vi "OneBallAuton.vi"   [LabVIEW 2013]
uses:
  <vilib>/Rock Robotics/WPI/SafetyOutput/WPI_SafetyOutputConfigMenu.ctl
  <vilib>/Rock Robotics/WPI/Solenoid/WPI_SolenoidValue.ctl
  <vilib>/Rock Robotics/WPI/RobotDrive/WPI_RobotDriveGetSetRefNum.vi
  <vilib>/Rock Robotics/WPI/Solenoid/WPI_SolenoidSetEnum.vi
types:
  T1 = typedef "WPI_SafetyOutputConfigMenu.ctl" = enum16{"Enable", "Disable"}
  T2 = typedef "WPI_RobotDriveDevRef.ctl" = cluster{"DevStatus":errorcluster, "Motors[]":T3[], "Square Inputs":bool, "Max Output":dbl, "Isochronous":bool}
  T3 = typedef "WPI_MotorControlDeviceRef.ctl" = cluster{"DeviceStatus":errorcluster, "Type":enum16{"PWM", "CAN"}, "PWM":cluster{"Digital Module":T4, "PWM Channel":T5, "DeadBand":T6}, "CAN":cluster{"Device Number":u8, "Control Mode":T7, "Semaphore":T8, "Max Vout":dbl}, "Invert":bool, "TransformRef":T9, "InvTransformRef":T9}
  T4 = typedef "FPGA_TypedefDigitalModule.ctl" = enum16{"Digital Module 1", "Digital Module 2"}
  T5 = typedef "FPGA_DIOPWMChannel.ctl" = enum8{"PWM 1", "PWM 2", "PWM 3", "PWM 4", "PWM 5", "PWM 6", "PWM 7", "PWM 8", "PWM 9", "PWM 10", "Invalid"}
  T6 = typedef "WPI_PWMDeadband.ctl" = cluster{"Name":string, "maxPositivePwm":i32, "minPositivePwm":i32, "centerPwm":i32, "maxNegativePwm":i32, "minNegativePwm":i32, "angularRange":u16}
  T7 = typedef "WPI_CANJaguar_ControlMode.ctl" = enum8{"Percent VBus", "Current", "Speed", "Position", "Voltage"}
  T8 = typedef "Semaphore RefNum" = refnum<k1>
  T9 = typedef "WPI_PWMTransform_ConPane.ctl" = refnum<vi>
  T10 = typedef "WPI_SolenoidDevRef.ctl" = cluster{"DevStatus":errorcluster, "Solenoid Module":T11, "Forward Solenoid Channel":T12, "Reverse Solenoid Channel":T12}
  T11 = typedef "FPGA_TypedefSolenoidModule.ctl" = enum16{"Solenoid Module 1", "Solenoid Module 2"}
  T12 = typedef "WPI_SolenoidChannel.ctl" = enum8{"Solenoid 1", "Solenoid 2", "Solenoid 3", "Solenoid 4", "Solenoid 5", "Solenoid 6", "Solenoid 7", "Solenoid 8", "Invalid"}
  T13 = typedef "WPI_DigitalInputDevRef.ctl" = cluster{"DevStatus":errorcluster, "DIO Channel":T14, "Digital Module":T4}
  T14 = typedef "FPGA_DIOChannel.ctl" = enum8{"DIO 1", "DIO 2", "DIO 3", "DIO 4", "DIO 5", "DIO 6", "DIO 7", "DIO 8", "DIO 9", "DIO 10", "DIO 11", "DIO 12", "DIO 13", "DIO 14", "Invalid"}
  T15 = typedef "WPI_EncoderDevRef.ctl" = cluster{"DevStatus":errorcluster, "EncoderIndex":T16, "CounterIndex":T17, "DistancePerCount":dbl, "Decoding Type":T18}
  T16 = typedef "FPGA_EncoderIdx.ctl" = enum8{"Enc 0", "Enc 1", "Enc 2", "Enc 3", "Invalid"}
  T17 = typedef "FPGA_CounterCtrSystemIndex.ctl" = enum8{"Ctr 0", "Ctr 1", "Ctr 2", "Ctr 3", "Ctr 4", "Ctr 5", "Ctr 6", "Ctr 7", "Invalid"}
  T18 = typedef "WPI_EncoderType.ctl" = enum16{"1x", "2x", "4x"}
  T19 = typedef "WPI_SolenoidValue.ctl" = enum16{"Off", "On", "Forward", "Reverse"}
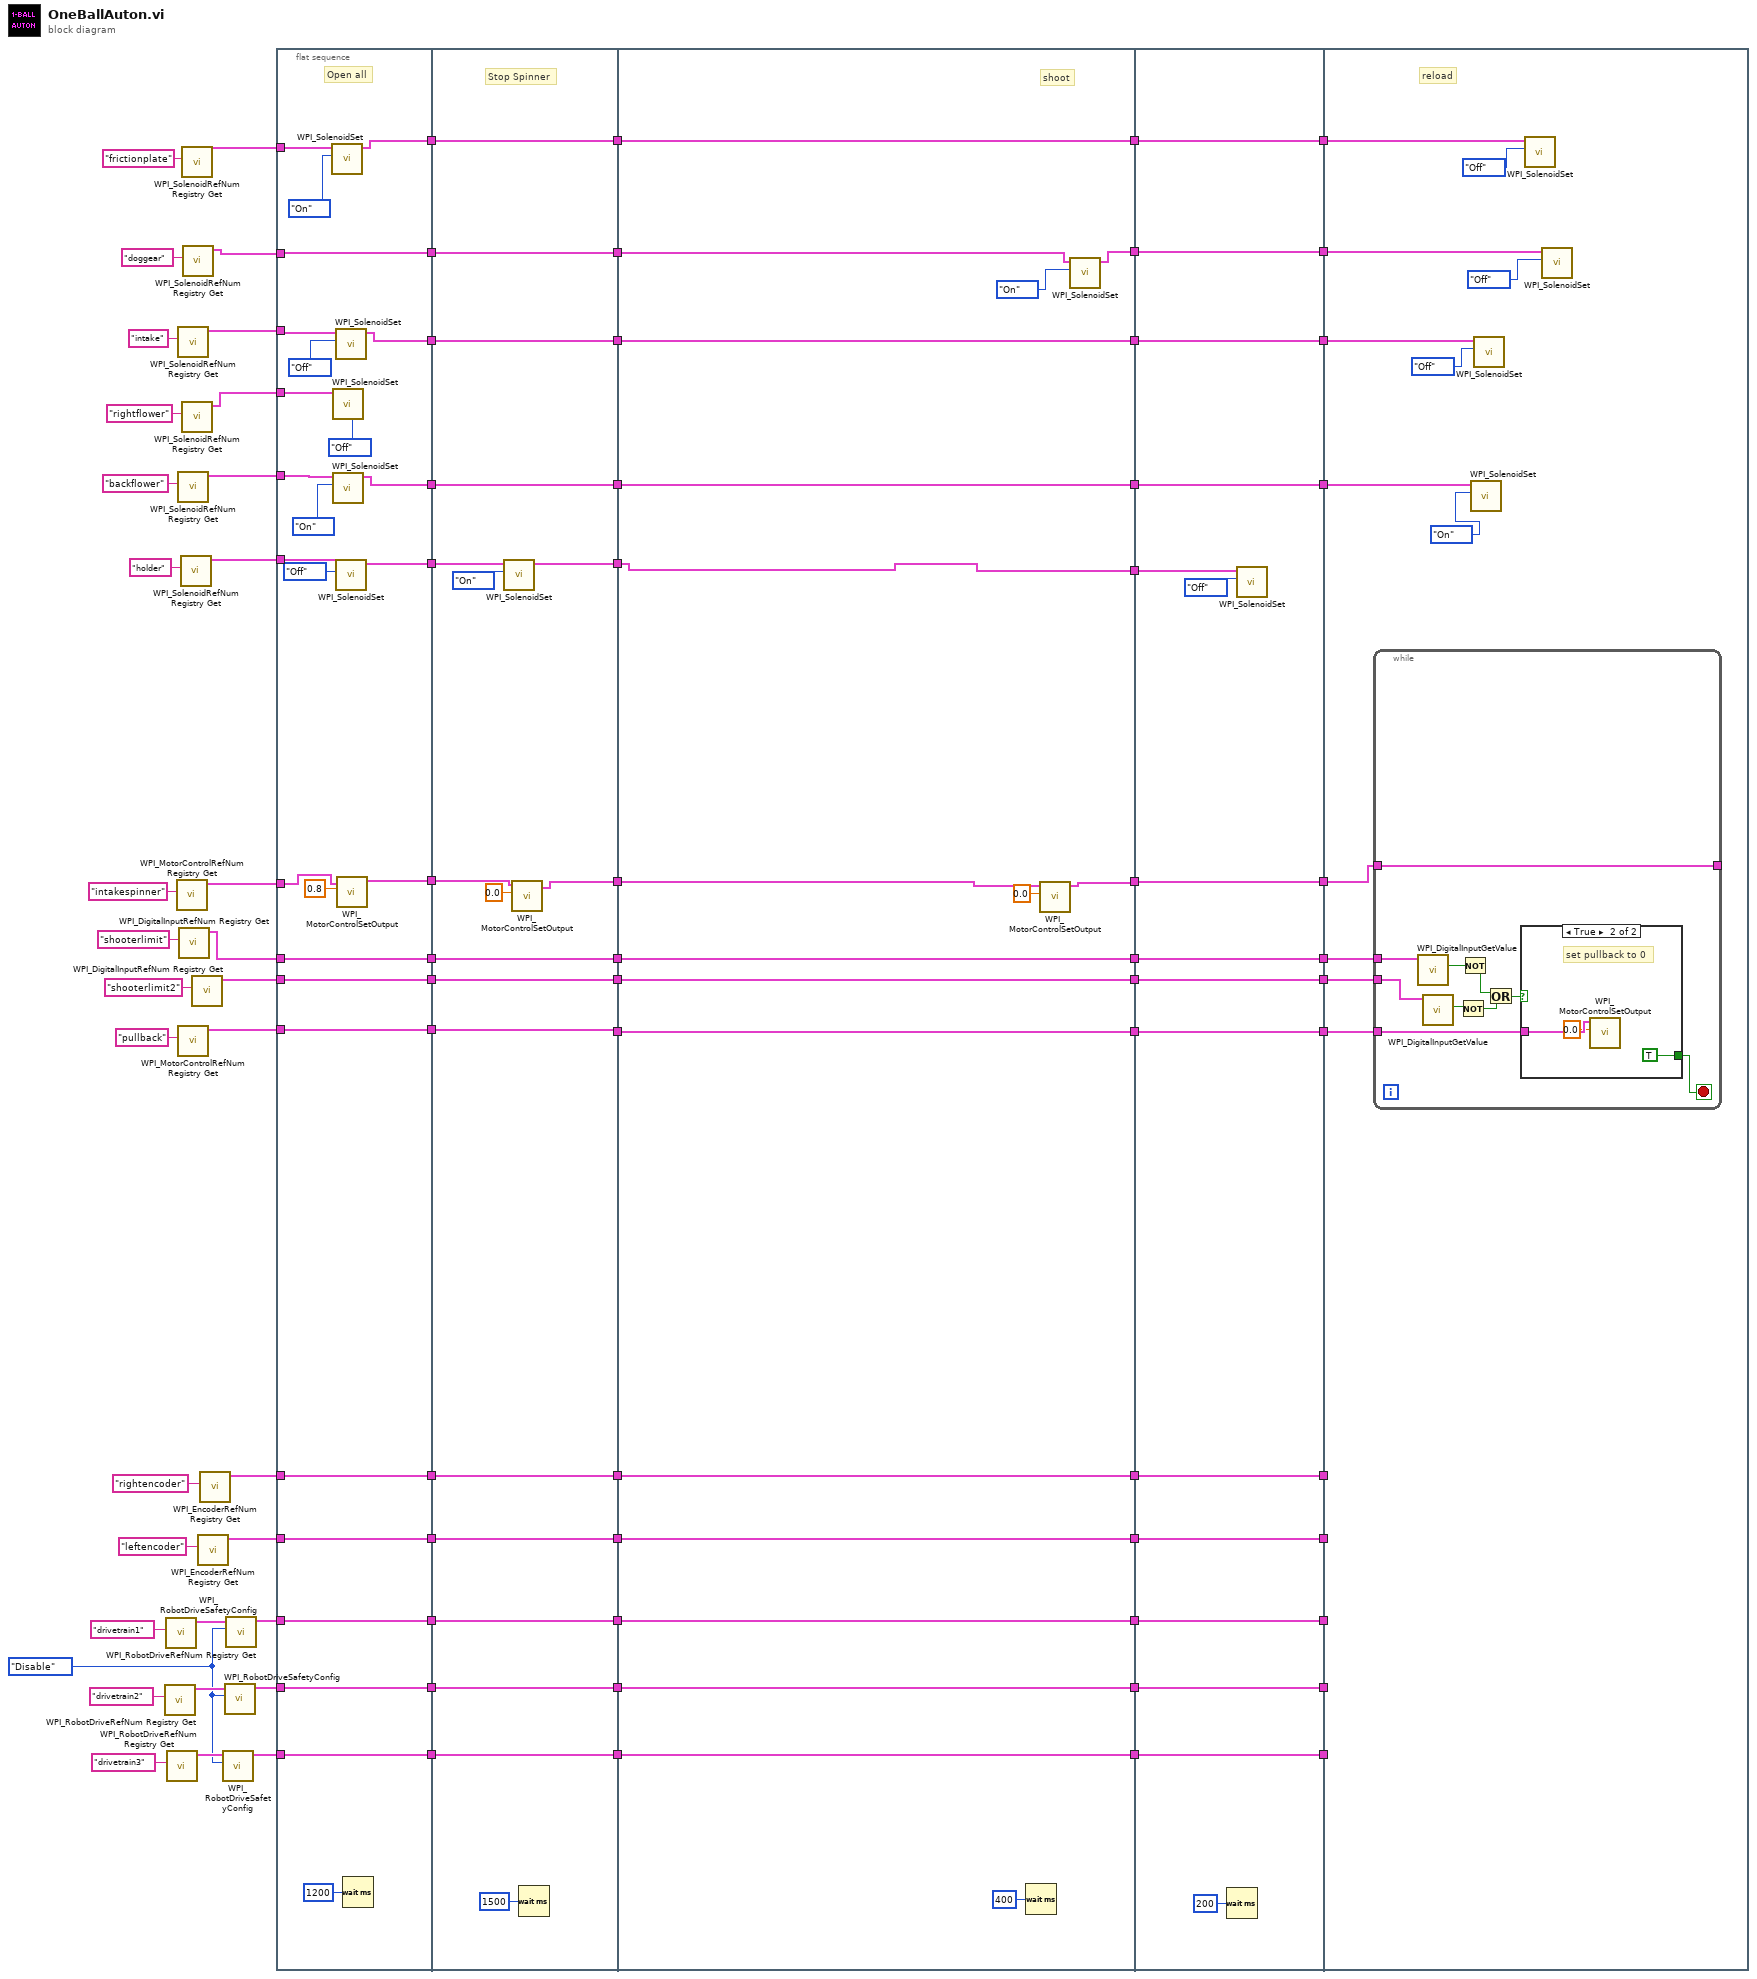
[diagram p0: block diagram]
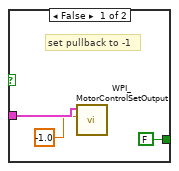
[diagram p2: hidden frame]
diagram:
  w58 = WPI_SafetyOutputConfigMenu."Disable" ("mode")
  n1 = call <vilib>:"WPI_RobotDriveRefNum Registry Get.vi"("refnum name"="drivetrain2") -> ("RobotDriveDevRef"=w60:T2)  [unwired: 9 in, 1 out]
  n2 = call <vilib>:"WPI_RobotDriveRefNum Registry Get.vi"("refnum name"="drivetrain1") -> ("RobotDriveDevRef"=w61:T2)  [unwired: 9 in, 1 out]
  n3 = call <vilib>:"WPI_RobotDriveRefNum Registry Get.vi"("refnum name"="drivetrain3") -> ("RobotDriveDevRef"=w59:T2)  [unwired: 9 in, 1 out]
  n4 = call <vilib>:"WPI_MotorControlRefNum Registry Get.vi"("refnum name"="intakespinner") -> ("MotorControlDevRef"=w71:T3)  [unwired: 9 in, 1 out]
  n5 = call <vilib>:"WPI_SolenoidRefNum Registry Get.vi"("refnum name"="intake") -> ("SolenoidDevRef"=w75:T10)  [unwired: 9 in, 1 out]
  n6 = call <vilib>:"WPI_SolenoidRefNum Registry Get.vi"("refnum name"="backflower") -> ("SolenoidDevRef"=w73:T10)  [unwired: 9 in, 1 out]
  n7 = call <vilib>:"WPI_MotorControlRefNum Registry Get.vi"("refnum name"="pullback") -> ("MotorControlDevRef"=w67:T3)  [unwired: 9 in, 1 out]
  n8 = call <vilib>:"WPI_DigitalInputRefNum Registry Get.vi"("refnum name"="shooterlimit") -> ("DigitalInputDevRef"=w69:T13)  [unwired: 9 in, 1 out]
  n9 = call <vilib>:"WPI_SolenoidRefNum Registry Get.vi"("refnum name"="holder") -> ("SolenoidDevRef"=w43:T10)  [unwired: 9 in, 1 out]
  n10 = call <vilib>:"WPI_SolenoidRefNum Registry Get.vi"("refnum name"="frictionplate") -> ("SolenoidDevRef"=w51:T10)  [unwired: 9 in, 1 out]
  n11 = call <vilib>:"WPI_SolenoidRefNum Registry Get.vi"("refnum name"="rightflower") -> ("SolenoidDevRef"=w74:T10)  [unwired: 9 in, 1 out]
  n12 = call <vilib>:"WPI_SolenoidRefNum Registry Get.vi"("refnum name"="doggear") -> ("SolenoidDevRef"=w79:T10)  [unwired: 9 in, 1 out]
  n13 = call <vilib>:"WPI_DigitalInputRefNum Registry Get.vi"("refnum name"="shooterlimit2") -> ("DigitalInputDevRef"=w46:T13)  [unwired: 9 in, 1 out]
  n14 = call <vilib>:"WPI_EncoderRefNum Registry Get.vi"("refnum name"="leftencoder") -> ("EncoderDevRef"=w56:T15)  [unwired: 9 in, 1 out]
  n15 = call <vilib>:"WPI_EncoderRefNum Registry Get.vi"("refnum name"="rightencoder") -> ("EncoderDevRef"=w57:T15)  [unwired: 9 in, 1 out]
  n16 = call <vilib>:"WPI_RobotDriveSafetyConfig.vi"("mode"=w58, "RobotDriveDevRef"=w59) -> ("RobotDriveDevRef"=w53:T2)  [unwired: 8 in, 1 out]
  n17 = call <vilib>:"WPI_RobotDriveSafetyConfig.vi"("mode"=w58, "RobotDriveDevRef"=w60) -> ("RobotDriveDevRef"=w54:T2)  [unwired: 8 in, 1 out]
  n18 = call <vilib>:"WPI_RobotDriveSafetyConfig.vi"("mode"=w58, "RobotDriveDevRef"=w61) -> ("RobotDriveDevRef"=w55:T2)  [unwired: 8 in, 1 out]
  n19 = flat-sequence {
    tunnel: w79 -> [w116]
    tunnel: [w116] -> w89
    tunnel: w75 -> [w115]
    tunnel: w74 -> [w114]
    tunnel: w73 -> [w113]
    tunnel: w71 -> [w111]
    tunnel: [w109] -> w88
    tunnel: w69 -> [w108]
    tunnel: [w108] -> w87
    tunnel: w67 -> [w107]
    tunnel: [w107] -> w86
    tunnel: [w106] -> w85
    tunnel: w57 -> [w106]
    tunnel: [w105] -> w84
    tunnel: w56 -> [w105]
    tunnel: [w104] -> w83
    tunnel: w55 -> [w104]
    tunnel: [w103] -> w82
    tunnel: w54 -> [w103]
    tunnel: [w102] -> w81
    tunnel: w53 -> [w102]
    tunnel: w51 -> [w99]
    tunnel: [w97] -> w50
    tunnel: [w96] -> w49
    tunnel: [w95] -> w48
    tunnel: w46 -> [w94]
    tunnel: [w94] -> w45
    tunnel: w43 -> [w93]
    tunnel: [w91] -> w42
    tunnel: w89 -> [w129]
    tunnel: w88 -> [w135]
    tunnel: [w132] -> w14
    tunnel: [w131] -> w13
    tunnel: w87 -> [w131]
    tunnel: w86 -> [w130]
    tunnel: [w130] -> w12
    tunnel: [w129] -> w11
    tunnel: w85 -> [w127]
    tunnel: w84 -> [w128]
    tunnel: [w128] -> w10
    tunnel: [w127] -> w9
    tunnel: w83 -> [w126]
    tunnel: w82 -> [w125]
    tunnel: [w126] -> w8
    tunnel: [w125] -> w7
    tunnel: w81 -> [w124]
    tunnel: [w124] -> w6
    tunnel: w50 -> [w123]
    tunnel: [w123] -> w5
    tunnel: [w122] -> w4
    tunnel: w49 -> [w122]
    tunnel: [w121] -> w3
    tunnel: w48 -> [w121]
    tunnel: w45 -> [w120]
    tunnel: [w120] -> w2
    tunnel: w42 -> [w119]
    tunnel: [w117] -> w1
    tunnel: [w151] -> w25
    tunnel: [w154] -> w27
    tunnel: [w153] -> w29
    tunnel: [w147] -> w31
    tunnel: [w145] -> w33
    tunnel: [w144] -> w35
    tunnel: [w143] -> w37
    tunnel: [w142] -> w39
    tunnel: [w141] -> w41
    tunnel: [w140] -> w23
    tunnel: [w139] -> w21
    tunnel: [w138] -> w19
    tunnel: [w137] -> w17
    tunnel: [w136] -> w15
    tunnel: w14 -> [w152]
    tunnel: w13 -> [w154]
    tunnel: w12 -> [w153]
    tunnel: w11 -> [w146]
    tunnel: w10 -> [w145]
    tunnel: w9 -> [w144]
    tunnel: w8 -> [w143]
    tunnel: w7 -> [w142]
    tunnel: w6 -> [w141]
    tunnel: w5 -> [w140]
    tunnel: w4 -> [w139]
    tunnel: w3 -> [w138]
    tunnel: w2 -> [w137]
    tunnel: w1 -> [w136]
    tunnel: w41 -> [w170]
    tunnel: [w170] -> w40
    tunnel: w39 -> [w169]
    tunnel: [w169] -> w38
    tunnel: w37 -> [w168]
    tunnel: [w168] -> w36
    tunnel: w35 -> [w167]
    tunnel: [w167] -> w34
    tunnel: w33 -> [w166]
    tunnel: [w166] -> w32
    tunnel: w31 -> [w165]
    tunnel: [w165] -> w30
    tunnel: w29 -> [w164]
    tunnel: [w164] -> w28
    tunnel: w27 -> [w163]
    tunnel: [w163] -> w26
    tunnel: w25 -> [w162]
    tunnel: [w162] -> w24
    tunnel: w23 -> [w161]
    tunnel: [w161] -> w22
    tunnel: w21 -> [w160]
    tunnel: [w160] -> w20
    tunnel: w19 -> [w159]
    tunnel: [w159] -> w18
    tunnel: w17 -> [w158]
    tunnel: [w158] -> w16
    tunnel: w15 -> [w155]
    tunnel: w40 -> [_]
    tunnel: w38 -> [_]
    tunnel: w36 -> [_]
    tunnel: w34 -> [_]
    tunnel: w32 -> [_]
    tunnel: w30 -> [w178]
    tunnel: w28 -> [w181]
    tunnel: w26 -> [w182]
    tunnel: w24 -> [w180]
    tunnel: w22 -> [w176]
    tunnel: w20 -> [w175]
    tunnel: w18 -> [w174]
    tunnel: w16 -> [w172]
    frame #0 {
      # "Open all"
      n20 = call-poly <vilib>:"WPI_SolenoidSet.vi"("Value"=WPI_SolenoidValue."On", "SolenoidDevRef"=w99) -> ("SolenoidDevRef"=w97:T10)  [unwired: 8 in, 1 out]
      n21 = call-poly <vilib>:"WPI_SolenoidSet.vi"("Value"=WPI_SolenoidValue."Off", "SolenoidDevRef"=w114) -> ()  [unwired: 8 in, 2 out]
      n22 = call-poly <vilib>:"WPI_SolenoidSet.vi"("Value"=WPI_SolenoidValue."On", "SolenoidDevRef"=w113) -> ("SolenoidDevRef"=w95:T10)  [unwired: 8 in, 1 out]
      n23 = call-poly <vilib>:"WPI_SolenoidSet.vi"("Value"=WPI_SolenoidValue."Off", "SolenoidDevRef"=w115) -> ("SolenoidDevRef"=w96:T10)  [unwired: 8 in, 1 out]
      n24 = call-poly <vilib>:"WPI_SolenoidSet.vi"("Value"=WPI_SolenoidValue."Off", "SolenoidDevRef"=w93) -> ("SolenoidDevRef"=w91:T10)  [unwired: 8 in, 1 out]
      n25 = call <vilib>:"WPI_MotorControlSetOutput.vi"("Output"=0.8, "MotorControlDevRef"=w111) -> ("MotorControlDevRef"=w109:T3)  [unwired: 7 in, 2 out]
      n26 = Wait (ms)(milliseconds to wait=u32 1200) -> ()  [unwired: 1 out]
    }
    frame #1 {
      # "Stop Spinner"
      n27 = call-poly <vilib>:"WPI_SolenoidSet.vi"("Value"=WPI_SolenoidValue."On", "SolenoidDevRef"=w119) -> ("SolenoidDevRef"=w117:T10)  [unwired: 8 in, 1 out]
      n28 = call <vilib>:"WPI_MotorControlSetOutput.vi"("Output"=0.0, "MotorControlDevRef"=w135) -> ("MotorControlDevRef"=w132:T3)  [unwired: 7 in, 2 out]
      n29 = Wait (ms)(milliseconds to wait=u32 1500) -> ()  [unwired: 1 out]
    }
    frame #2 {
      # "shoot"
      n30 = Wait (ms)(milliseconds to wait=u32 400) -> ()  [unwired: 1 out]
      n31 = call <vilib>:"WPI_MotorControlSetOutput.vi"("Output"=0.0, "MotorControlDevRef"=w152) -> ("MotorControlDevRef"=w151:T3)  [unwired: 7 in, 2 out]
      n32 = call-poly <vilib>:"WPI_SolenoidSet.vi"("Value"=WPI_SolenoidValue."On", "SolenoidDevRef"=w146) -> ("SolenoidDevRef"=w147:T10)  [unwired: 8 in, 1 out]
    }
    frame #3 {
      n33 = Wait (ms)(milliseconds to wait=u32 200) -> ()  [unwired: 1 out]
      n34 = call-poly <vilib>:"WPI_SolenoidSet.vi"("Value"=WPI_SolenoidValue."Off", "SolenoidDevRef"=w155) -> ()  [unwired: 8 in, 2 out]
    }
    frame #4 {
      # "reload"
      n35 = while {
        tunnel: w182 -> [w192]
        tunnel: w181 -> [w190]
        tunnel: [w188] -> _
        tunnel: w180 -> [w188]
        tunnel: w172 -> [w187]
        stop <- w189 stop-if-true
        n36 = call <vilib>:"WPI_DigitalInputGetValue.vi"("DigitalInputDevRef"=w192) -> ("Value"=w191:bool)  [unwired: 8 in, 2 out]
        n37 = call <vilib>:"WPI_DigitalInputGetValue.vi"("DigitalInputDevRef"=w187) -> ("Value"=w183:bool)  [unwired: 8 in, 2 out]
        n38 = Not(x=w183) -> (.not. x?=w184:bool)
        n39 = Not(x=w191) -> (.not. x?=w186:bool)
        n40 = Or(x=w186, y=w184) -> (x .or. y?=w185:bool)
        n41 = case shown="True" w185 {
          tunnel: w190 -> [w195 w198]
          tunnel: [FALSE TRUE] -> w189
          frame False {
            # "set pullback to -1"
            n42 = call <vilib>:"WPI_MotorControlSetOutput.vi"("Output"=-1.0, "MotorControlDevRef"=w195) -> ()  [unwired: 7 in, 3 out]
          }
          frame True {
            # "set pullback to 0"
            n43 = call <vilib>:"WPI_MotorControlSetOutput.vi"("Output"=0.0, "MotorControlDevRef"=w198) -> ()  [unwired: 7 in, 3 out]
          }
        }
      }
      n44 = call-poly <vilib>:"WPI_SolenoidSet.vi"("Value"=WPI_SolenoidValue."On", "SolenoidDevRef"=w174) -> ()  [unwired: 8 in, 2 out]
      n45 = call-poly <vilib>:"WPI_SolenoidSet.vi"("Value"=WPI_SolenoidValue."Off", "SolenoidDevRef"=w175) -> ()  [unwired: 8 in, 2 out]
      n46 = call-poly <vilib>:"WPI_SolenoidSet.vi"("Value"=WPI_SolenoidValue."Off", "SolenoidDevRef"=w176) -> ()  [unwired: 8 in, 2 out]
      n47 = call-poly <vilib>:"WPI_SolenoidSet.vi"("Value"=WPI_SolenoidValue."Off", "SolenoidDevRef"=w178) -> ()  [unwired: 8 in, 2 out]
    }
  }
